vi "Read Upper Voltage Limit.vi"(8 "error in (no error)":errorcluster, 11 "VISA resource name":refnum<visa-resource-name>) -> (0 "error out":errorcluster, 2 "OVP":dbl format="%.1g", 3 "VISA resource name out":refnum<visa-resource-name>)   [LabVIEW 2021, in "BK Precision 169XB.lvlib"]
doc: "Returns the actual voltage level and actual current level for a desired channel."
uses:
  BK Precision 169XB.lvlib
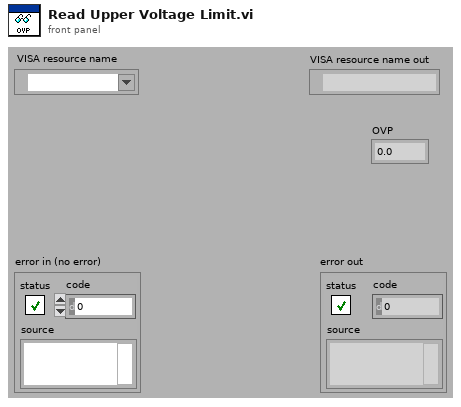
[diagram p1: front panel]
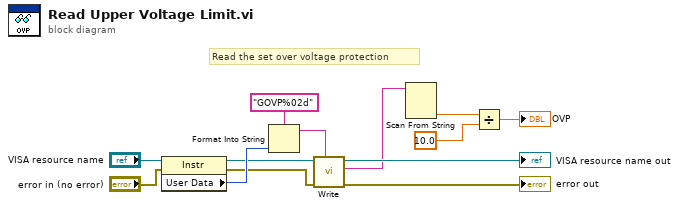
[diagram p0: block diagram]
diagram:
  # "Read the set over voltage protection"
  n1 = property class="Instr"(reference="VISA resource name", error in="error in (no error)") -> (reference out=w3:refnum<visa-resource-name>, error out=w2:errorcluster, "User Data"=w6:u32)
  n2 = Format Into String(format string="GOVP%02d", w6) -> (resulting string=w1:string)  [unwired: 2 in, 1 out]
  n3 = call "Write.vi"("Input String"=w1, "error in (no error)"=w2, "VISA resource name"=w3) -> ("error out"=→"error out":errorcluster, "String"=w8:string, "VISA resource name out"=→"VISA resource name out":refnum<visa-resource-name>)  [unwired: 6 in]
  n4 = Scan From String(input string=w8) -> (output 1=w13:dbl)  [unwired: 4 in, 3 out]
  n5 = Divide(x=w13, y=10.0) -> (x/y=→"OVP":dbl)
